vi "Recursive List.vi"(8 "error in (no error)":errorcluster, 11 "Runnable in":refnum<class "Runnable.lvclass">) -> (0 "error out":errorcluster, 3 "List of Runnables":string[](array[string]))   [LabVIEW 2020, in "LUnit Test Suite.lvclass"]
uses:
  LUnit Test Suite.lvclass
  LUnit Test Suite.lvclass/LUnit Test Suite.ctl
  Runnable/Runnable.lvclass
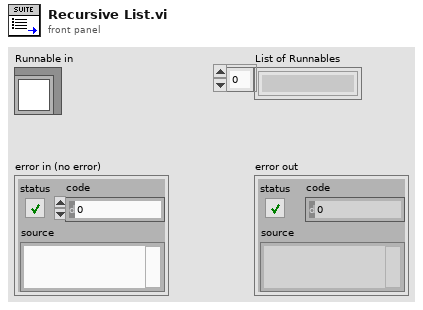
[diagram p1: front panel]
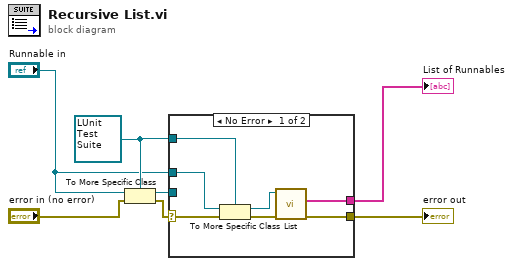
[diagram p0: block diagram]
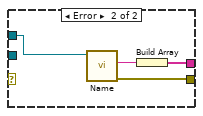
[diagram p2: hidden frame]
diagram:
  w7 = refnum<class "LUnit Test Suite.lvclass"> refnum ("LUnit Test Suite.lvclass")
  n1 = To More Specific Class(target class=w7, reference="Runnable in", error in="error in (no error)") -> (specific class reference=w3:refnum<class "LUnit Test Suite.lvclass">, error out=w4:errorcluster)
  n2 = case shown="No Error" w4 {
    selector: w4 -> [w10 _]
    tunnel: [w14 w16] -> w1
    tunnel: [w13 w15] -> w2
    tunnel: w3 -> [_ _]
    tunnel: "Runnable in" -> [w12 w18]
    tunnel: w7 -> [w11 _]
    frame No Error {
      n3 = To More Specific Class(target class=w11, reference=w12, error in=w10) -> (specific class reference=w8:refnum<class "LUnit Test Suite.lvclass">, error out=w9:errorcluster)
      n4 = call "List.vi"("error in (no error)"=w9, "LUnit Test Suite In"=w8) -> ("error out"=w13:errorcluster, "List of Runnables"=w14:string[])  [unwired: 8 in]
    }
    frame Error {
      n5 = call-dynamic "Name.vi"("Runnable in"=w18) -> ("error out"=w15:errorcluster, "Name"=w17:string)  [unwired: 8 in, 1 out]
      n6 = Build Array(w17) -> (w16:string[])
    }
  }
  "error out" <- w2
  "List of Runnables" <- w1
